vi "Instance History.vi"(0 "Instance Data Array in":T1[](array[typedef]), 1 "Selected Instance":string, 2 "Class Data":refnum<class "Arithemetic Operation.lvclass">, 3 "Error In":errorcluster, 4 "Delete?":bool) -> (7 "Instance Data Array out":T1[](array[typedef]), 10 "Error Out":errorcluster)   [LabVIEW 2019, in "Arithemetic Operation.lvclass"]
uses:
  Arithemetic Operation.lvclass
  Typedef/Class Data.ctl
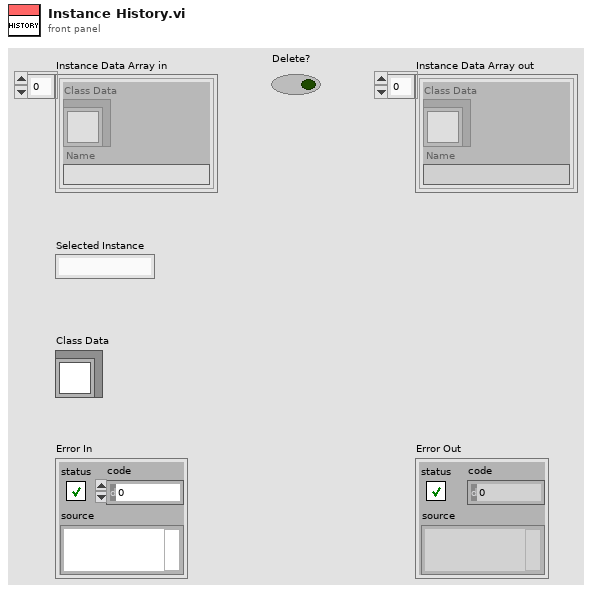
[diagram p1: front panel]
types:
  T1 = typedef "Class Data.ctl" = cluster{"Class Data":refnum<class "Arithemetic Operation.lvclass">, "Name":string}
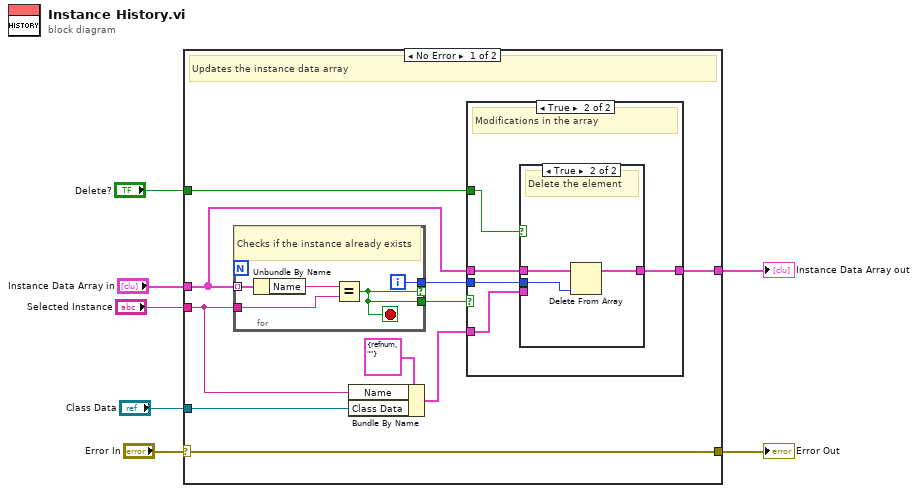
[diagram p0: block diagram]
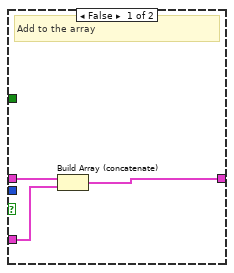
[diagram p2: hidden frame]
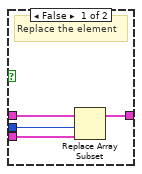
[diagram p3: hidden frame]
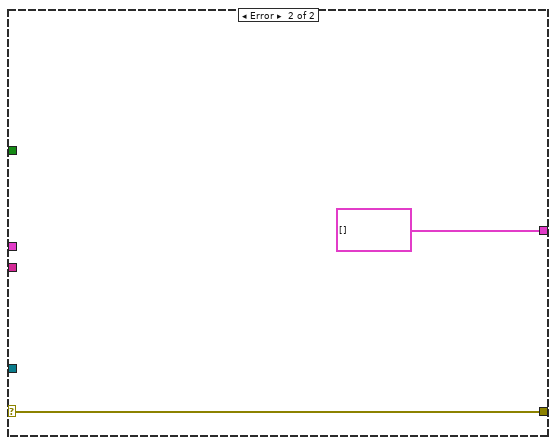
[diagram p4: hidden frame]
diagram:
  n1 = case shown="No Error" "Error In" {
    selector: "Error In" -> [w17 w39]
    tunnel: [w17 w39] -> w6
    tunnel: [w12 T1[] [] ("Instance Data Array in")] -> w5
    tunnel: "Class Data" -> [w11 _]
    tunnel: "Selected Instance" -> [w10 _]
    tunnel: "Instance Data Array in" -> [w9 _]
    tunnel: "Delete?" -> [w8 _]
    frame No Error {
      # "Updates the instance data array"
      n2 = for {
        tunnel: w9 -> [w37] mode=indexing
        tunnel: w10 -> [w35]
        tunnel: [w34] -> w15 if=w33
        tunnel: [w33] -> w14
        i -> [w34]
        stop <- w33 stop-if-true
        # "Checks if the instance already exists"
        n3 = Unbundle By Name(w37) -> ("Name"=w36:string)
        n4 = Equal?(x=w36, y=w35) -> (x = y?=w33:bool)
      }
      n5 = Bundle By Name(cluster=T1 {"Class Data"=refnum, "Name"=""}, "Name"=w10, "Class Data"=w11) -> (w16:T1)
      n6 = case shown="True" w14 {
        tunnel: w15 -> [_ w25]
        tunnel: w9 -> [w20 w24]
        tunnel: w16 -> [w19 w22]
        tunnel: [w18 w23] -> w12
        tunnel: w8 -> [_ w21]
        frame False {
          # "Add to the array"
          n7 = Build Array (concatenate)(w20, w19) -> (w18:T1[])
        }
        frame True {
          # "Modifications in the array"
          n8 = case shown="True" w21 {
            tunnel: w25 -> [w29 w30]
            tunnel: w24 -> [w28 w32]
            tunnel: [w27 w31] -> w23
            tunnel: w22 -> [w26 _]
            frame False {
              # "Replace the element"
              n9 = Replace Array Subset(array=w28, new element=w26, index=w29) -> (w27:T1[])
            }
            frame True {
              # "Delete the element"
              n10 = Delete From Array(array=w32, index=w30) -> (array with subset deleted=w31:T1[])  [unwired: 1 in, 1 out]
            }
          }
        }
      }
    }
    frame Error {
    }
  }
  "Error Out" <- w6
  "Instance Data Array out" <- w5
